vi "read csi and samples (host).vi"(0 "input cluster":T1 {"Daughterboard Clock Rate" format="%#.3pHz"; "FPGA Data Clock Rate" format="%#.3pHz"; "Data Clock Rate" format="%#.3pHz"; "Characterization Data"."Frequencies [Hz]" format="%#_6p"; "EEPROM Characterization Header"."Pointer to Device Data Header" format="%x"; "EEPROM Characterization Header"."Checksum" format="%x"; "Device Data Header"."Pointer to Characterization Data" format="%x"; "Device Data Header"."Checksum" format="%x"; "EEPROM Header"."Pointer to User Header" format="%x"; "EEPROM Header"."Pointer to Factory Header" format="%x"; "EEPROM Header"."Product Code" format="%x"; "EEPROM Header"."Checksum" format="%x"}, 5 "csi num":u32=1000, 9 "samples num":u32=1000, 11 "SNR threshold":dbl) -> (1 "signal power":dbl, 2 "noise power":dbl, 3 "CSI Remaining":u32, 4 "Power measurements Remaining":u32, 6 "csi":cdb[](array[numeric]), 10 "samples":cdb[](array[numeric]), 13 "SNR":dbl, 14 "samples remaining":u32, 15 "packet valid":bool)   [LabVIEW 2020]
uses:
  <instrlib>/niUsrpRio/Config/v1/Host/Public/niUsrpRio Session.ctl
  <instrlib>/_niInstr/Register Bus/v0/Host/Public/Register Bus Session.ctl
  <instrlib>/_niInstr/Register Bus/v0/Host/Private/Session Data.ctl
  <instrlib>/niUsrpRio/Config/v1/Host/Private/DB Queue Reference.ctl
  <instrlib>/niUsrpRio/Config/v1/Host/Private/Daughterboard Data.ctl
  <instrlib>/niUsrpRio/Config/v1/Host/Private/ATR state data.ctl
  <instrlib>/niUsrpRio/Config/v1/Host/Private/Antenna Configuration.ctl
  <instrlib>/niUsrpRio/Config/v1/Host/Private/CPLD Power Mode.ctl
  <instrlib>/niUsrpRio/Config/v1/Host/Public/EEPROM Header.ctl
  <instrlib>/niUsrpRio/Config/v1/Host/Public/EEPROM Device Data Header.ctl
  <instrlib>/niUsrpRio/Config/v1/Host/Public/EEPROM Characterization Header.ctl
  <instrlib>/niUsrpRio/Config/v1/Host/Public/Characterization Data.ctl
  <instrlib>/niUsrpRio/Config/v1/Host/Public/IQ Imbalance.ctl
  Host/SubVIs/Streaming Xvcr FPGA Ref.ctl
  <vilib>/Utility/error.llb/Error Cluster From Error Code.vi
  <vilib>/rvi/errors/niLvFpgaAdjustHostInterfaceError.vi
  <vilib>/rvi/interface/nirviMethod/nirviMethod.xnode
  <vilib>/FPGAPlugInAG/Dynamic/niLvFpga_ReadFifo_Dynamic.vi
  <vilib>/rvi/errors/niLvFpgaMergeErrorWithErrorCode.vi
  <instrlib>/_niInstr/Register Bus/v0/Host/niInstr Register Bus v0 Host.lvlib
  <instrlib>/niUsrpRio/Config/v1/Host/niUsrpRio Config v1 Host.lvlib
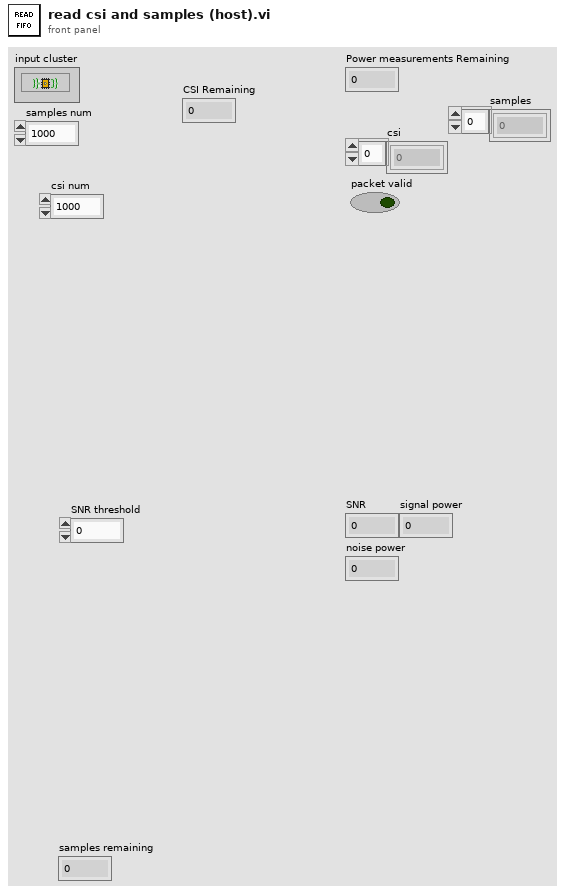
[diagram p1: front panel]
types:
  T1 = typedef "niUsrpRio Config v1 Host.lvlib/niUsrpRio Session.ctl" = cluster{"FPGA Interface":refnum<k20>, "RIO Interface Number":u32, "Data Clock Rate":u32, "FPGA Data Clock Rate":u32, "Global Settings Register Bus":T2, "Radio 0 Settings Register Bus":T2, "Radio 1 Settings Register Bus":T2, "Radio Settings Bus Semaphore":T3, "DB Queues":T4[], "Characterization Data Valid?":bool, "EEPROM Header":T5, "Device Data Header":T6, "EEPROM Characterization Header":T7, "Characterization Data":T8[], "FPGA Current Version":u32, "FPGA Oldest Compatible Version":u32, "Fixed Logic Current Version":u32, "Fixed Logic Oldest Compatible Version":u32, "FPGA Radio Settings Bus Current Version":u32, "FPGA Radio Settings Bus Oldest Compatible Version":u32, "FPGA Board Config Current Version":u32, "FPGA Board Config Oldest Compatible Version":u32, "Daughterboard Clock Rate":u32, "daughterboard configuration session handles":u64[]}
  T2 = typedef "niInstr Register Bus v0 Host.lvlib/Register Bus Session.ctl" = refnum<queue>
  T3 = typedef "Semaphore RefNum" = refnum<k1>
  T4 = typedef "niUsrpRio Config v1 Host.lvlib/DB Queue Reference.ctl" = refnum<queue>
  T5 = typedef "niUsrpRio Config v1 Host.lvlib/EEPROM Header.ctl" = cluster{"Checksum":u32, "Product Code":u16, "Hardware Current Version":u16, "Hardware Oldest Compatible Version":u16, "EEPROM Map Current Version":u16, "EEPROM Map Oldest Compatible Version":u16, "User Password":string, "Pointer to Factory Header":u32, "Pointer to User Header":u32, "Recommended Interval":u16, "Number of Reserved Bytes":i32, "Number of Daughterboards":u8, "Daughterboard IDs":u16[], "Daughterboard Serial Numbers":string[]}
  T6 = typedef "niUsrpRio Config v1 Host.lvlib/EEPROM Device Data Header.ctl" = cluster{"Checksum":u32, "Number of Channels":u8, "Number of Gain Settings":u16[], "Pointer to Characterization Data":u32[], "Number of Reserved Bytes":i32, "Number of Frequencies":u16[]}
  T7 = typedef "niUsrpRio Config v1 Host.lvlib/EEPROM Characterization Header.ctl" = cluster{"Checksum":u32, "Date":timestamp, "Temperature":sgl, "Misc. Info":string, "Pointer to Device Data Header":u32, "Number of Reserved Bytes":i32}
  T8 = typedef "niUsrpRio Config v1 Host.lvlib/Characterization Data.ctl" = cluster{"Gains[dB]":dbl[], "Frequencies [Hz]":dbl[], "IQ Imbalance Table":T9[], "Measured Gains[dB]":dbl[][]}
  T9 = typedef "niUsrpRio Config v1 Host.lvlib/IQ Imbalance.ctl" = cluster{"Gain Imbalance [linear]":dbl, "Phase Imbalance [radians]":dbl, "Offset":cdb}
  T10 = typedef "Streaming Xvcr FPGA Ref.ctl" = refnum<k20>
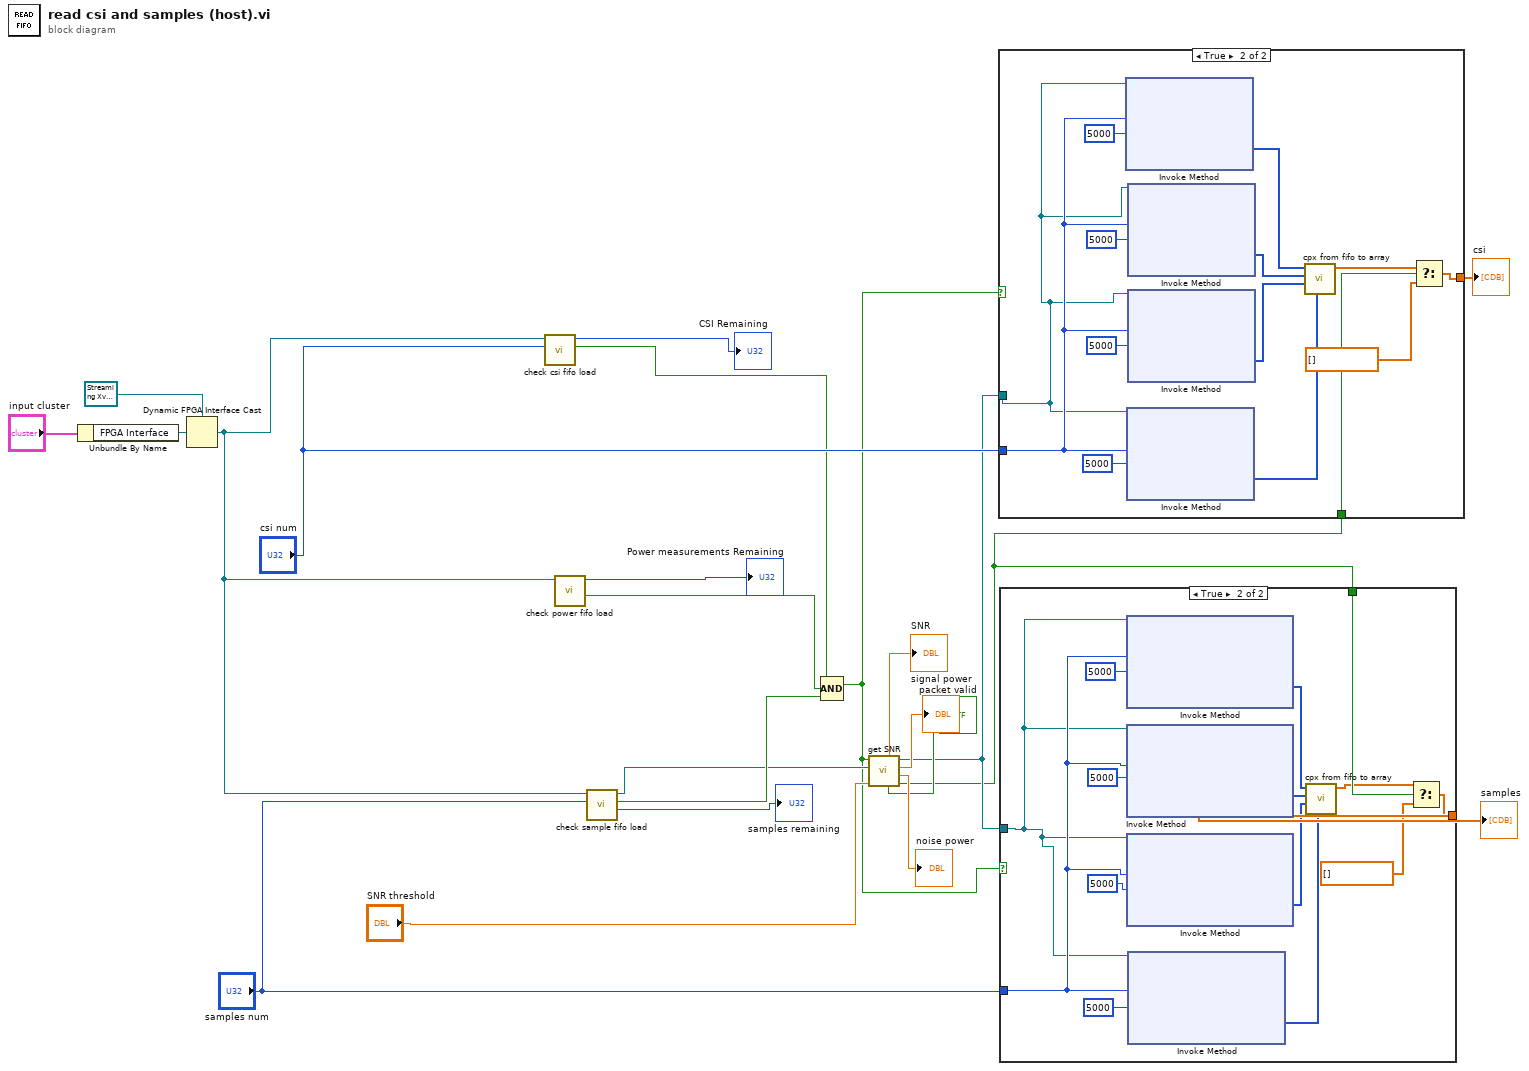
[diagram p0: block diagram]
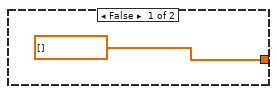
[diagram p2: hidden frame]
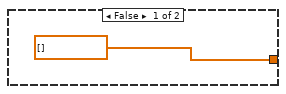
[diagram p3: hidden frame]
diagram:
  n1 = Unbundle By Name("input cluster") -> ("FPGA Interface"=w21:refnum<k20>)
  n2 = Dynamic FPGA Interface Cast(Session In=T10 refnum ("Type"), Type=w21) -> (Session Out=w8:T10)
  n3 = call "check csi fifo load.vi"("csi num"="csi num", "Refnum in"=w8) -> ("Boolean"=w17:bool, "CSI Remaining"=→"CSI Remaining":u32)  [unwired: 8 in]
  n4 = call "check power fifo load.vi"("Refnum in"=w8) -> ("ready"=w16:bool, "Power measurements Remaining"=→"Power measurements Remaining":u32)  [unwired: 9 in]
  n5 = call "check sample fifo load.vi"("samples num"="samples num", "Refnum in"=w8) -> ("samples remaining"=→"samples remaining":u32, "Boolean"=w15:bool, "Refnum out"=w13:T10)  [unwired: 7 in]
  n6 = Compound Arithmetic op=AND(w17, w16, w15) -> (w1:bool)
  n7 = call "get SNR.vi"("SNR threshold"="SNR threshold", "Refnum in"=w13, "fifo ready"=w1) -> ("packet valid now"=w2:bool, "noise power"=→"noise power":dbl, "signal power"=→"signal power":dbl, "FPGA VI Reference Out"=w3:T10, "packet valid"=→"packet valid":bool, "SNR"=→"SNR":dbl)  [unwired: 3 in]
  n8 = case shown="True" w1 {
    tunnel: "csi num" -> [_ w30]
    tunnel: w3 -> [_ w29]
    tunnel: [cdb[] [] w25] -> w19
    tunnel: w2 -> [_ w27]
    frame False {
    }
    frame True {
      n9 = xnode "Invoke Method"("FPGA VI Reference In"=w29, "Number of Elements"=w30, "Timeout (ms)"=5000) -> ("Data"=w33:u64[])  [unwired: 1 in, 3 out]
      n10 = xnode "Invoke Method"("FPGA VI Reference In"=w29, "Number of Elements"=w30, "Timeout (ms)"=5000) -> ("Data"=w38:u64[])  [unwired: 1 in, 3 out]
      n11 = xnode "Invoke Method"("FPGA VI Reference In"=w29, "Number of Elements"=w30, "Timeout (ms)"=5000) -> ("Data"=w32:u64[])  [unwired: 1 in, 3 out]
      n12 = xnode "Invoke Method"("FPGA VI Reference In"=w29, "Number of Elements"=w30, "Timeout (ms)"=5000) -> ("Data"=w31:u64[])  [unwired: 1 in, 3 out]
      n13 = call "cpx from fifo to array.vi"("channel 1"=w38, "channel 2"=w31, "channel 3"=w32, "channel 4"=w33) -> ("Array"=w28:cdb[])  [unwired: 7 in]
      n14 = Select(t=w28, s=w27, f=cdb[] []) -> (s? t:f=w25:cdb[])
    }
  }
  "csi" <- w19
  n15 = case shown="True" w1 {
    tunnel: "samples num" -> [_ w45]
    tunnel: w3 -> [_ w44]
    tunnel: [cdb[] [] w42] -> w14
    tunnel: w2 -> [_ w43]
    frame False {
    }
    frame True {
      n16 = xnode "Invoke Method"("FPGA VI Reference In"=w44, "Number of Elements"=w45, "Timeout (ms)"=5000) -> ("Data"=w48:u64[])  [unwired: 1 in, 3 out]
      n17 = xnode "Invoke Method"("FPGA VI Reference In"=w44, "Number of Elements"=w45, "Timeout (ms)"=5000) -> ("Data"=w47:u64[])  [unwired: 1 in, 3 out]
      n18 = xnode "Invoke Method"("FPGA VI Reference In"=w44, "Number of Elements"=w45, "Timeout (ms)"=5000) -> ("Data"=w46:u64[])  [unwired: 1 in, 3 out]
      n19 = xnode "Invoke Method"("FPGA VI Reference In"=w44, "Number of Elements"=w45, "Timeout (ms)"=5000) -> ("Data"=w53:u64[])  [unwired: 1 in, 3 out]
      n20 = call "cpx from fifo to array.vi"("channel 1"=w53, "channel 2"=w46, "channel 3"=w47, "channel 4"=w48) -> ("Array"=w41:cdb[])  [unwired: 7 in]
      n21 = Select(t=w41, s=w43, f=cdb[] []) -> (s? t:f=w42:cdb[])
    }
  }
  "samples" <- w14
